vi "Wait For Acquisition Complete.vi"(8 "error in (no error)":errorcluster, 10 "Maximum Time (10000)":u32=10000, 11 "VISA resource name":refnum<visa-resource-name>) -> (0 "error out":errorcluster, 3 "VISA resource name out":refnum<visa-resource-name>)   [LabVIEW 2011, in "Agilent E5052X.lvlib"]
doc: "Waits for the current sweep to finish. This VI should be called after Initiate VI and before Fetch Trace VI.\n\n<B>Note:</B> \n\nUse this VI only with other low-level VIs. The high-level VIs automatically incorporate this functionality. This VI does not check the instrument status."
uses:
  Agilent E5052X.lvlib
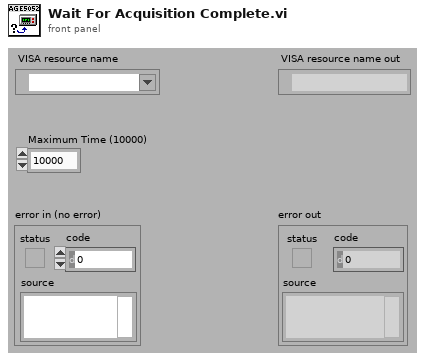
[diagram p1: front panel]
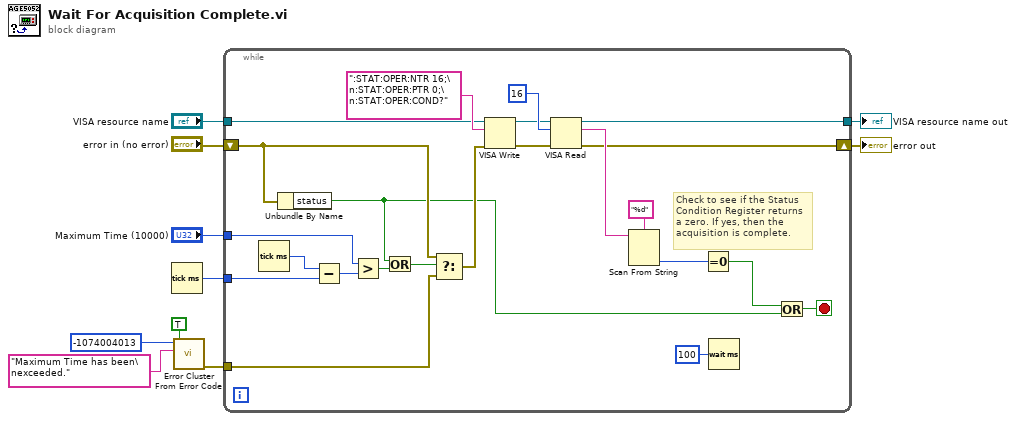
[diagram p0: block diagram]
diagram:
  n1 = Tick Count (ms)() -> (millisecond timer value=w5:u32)
  n2 = call <vilib>:"Error Cluster From Error Code.vi"("show call chain? (False)"=TRUE, "error message (\"\")"="Maximum Time has been\nexceeded." ("error message (\"\")"), "error code (0)"=-1074004013) -> ("error out"=w1:errorcluster)  [unwired: 6 in]
  n3 = while {
    tunnel: [w30] -> w9
    tunnel: "VISA resource name" -> [w27]
    tunnel: "Maximum Time (10000)" -> [w21]
    tunnel: w5 -> [w22]
    shift-right: [w31] -> w10
    shift-left: "error in (no error)" -> [w17]
    tunnel: w1 -> [w15]
    stop <- w20 stop-if-true
    # "Check to see if the Status Condition Register returns a zero. If yes, then the acquisition is complete."
    n4 = Tick Count (ms)() -> (millisecond timer value=w24:u32)
    n5 = Unbundle By Name(w17) -> ("status"=w14:bool)
    n6 = Subtract(x=w24, y=w22) -> (x-y=w23:u32)
    n7 = Greater?(x=w21, y=w23) -> (0:w18:bool)
    n8 = Or(x=w14, y=w18) -> (x .or. y?=w19:bool)
    n9 = Select(t=w17, s=w19, f=w15) -> (s? t:f=w16:errorcluster)
    n10 = VISA Write(VISA resource name=w27, write buffer=":STAT:OPER:NTR 16;\n:STAT:OPER:PTR 0;\n:STAT:OPER:COND?", error in (no error)=w16) -> (VISA resource name out=w25:refnum<visa-resource-name>, error out=w26:errorcluster)  [unwired: 1 out]
    n11 = VISA Read(VISA resource name=w25, byte count=u32 16, error in (no error)=w26) -> (VISA resource name out=w30:refnum<visa-resource-name>, read buffer=w33:string, error out=w31:errorcluster)  [unwired: 1 out]
    n12 = Scan From String(format string="%d", input string=w33) -> (output 1=w13:i32)  [unwired: 3 in, 3 out]
    n13 = Equal To 0?(x=w13) -> (x = 0?=w12:bool)
    n14 = Wait (ms)(milliseconds to wait=u32 100) -> ()  [unwired: 1 out]
    n15 = Or(x=w12, y=w14) -> (x .or. y?=w20:bool)
  }
  "error out" <- w10
  "VISA resource name out" <- w9
